vi "MecaKinematics_SetInverseKinematics.vi"(8 "RearRight":T2 {"Y" format="%14.3f"; "X" format="%14.3f"}, 9 "RearLeft":T2 {"Y" format="%14.3f"; "X" format="%14.3f"}, 10 "FrontRight":T2 {"Y" format="%14.3f"; "X" format="%14.3f"}, 11 "FrontLeft":T2 {"Y" format="%14.3f"; "X" format="%14.3f"}) -> (3 "InverseKinematics":T1)   [LabVIEW 2019, in "Trajectory_Library.lvlib"]
doc: "Construct inverse kinematics matrix from wheel locations.\n\nParameters:\n - FrontLeft - The location of the front-left wheel relative to the physical center of the robot.\n - FrontRight - The location of the front-right wheel relative to the physical center of the robot.\n - RearLeft - The location of the rear-left wheel relative to the physical center of the robot.\n - RearRight - The location of the rear-right wheel relative to the physical center of the robot.\n\nReturns:\n - InverseKinematics - Return matix"
uses:
  Trajectory_Library.lvlib
  TRANSLATION2D.ctl
  <vilib>/Analysis/Matrix/Datatypes/RealMatrix.ctl
  MatrixHelper_CoerceSize.vi
  <vilib>/Analysis/Matrix/NI_Matrix.lvlib
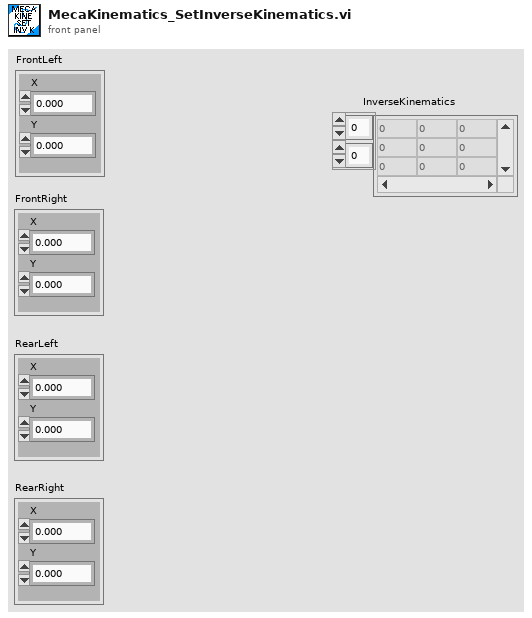
[diagram p1: front panel]
types:
  T1 = typedef "NI_Matrix.lvlib/RealMatrix.ctl" = dbl[][]
  T2 = typedef "Trajectory_Library.lvlib/TRANSLATION2D.ctl" = cluster{"X":dbl, "Y":dbl}
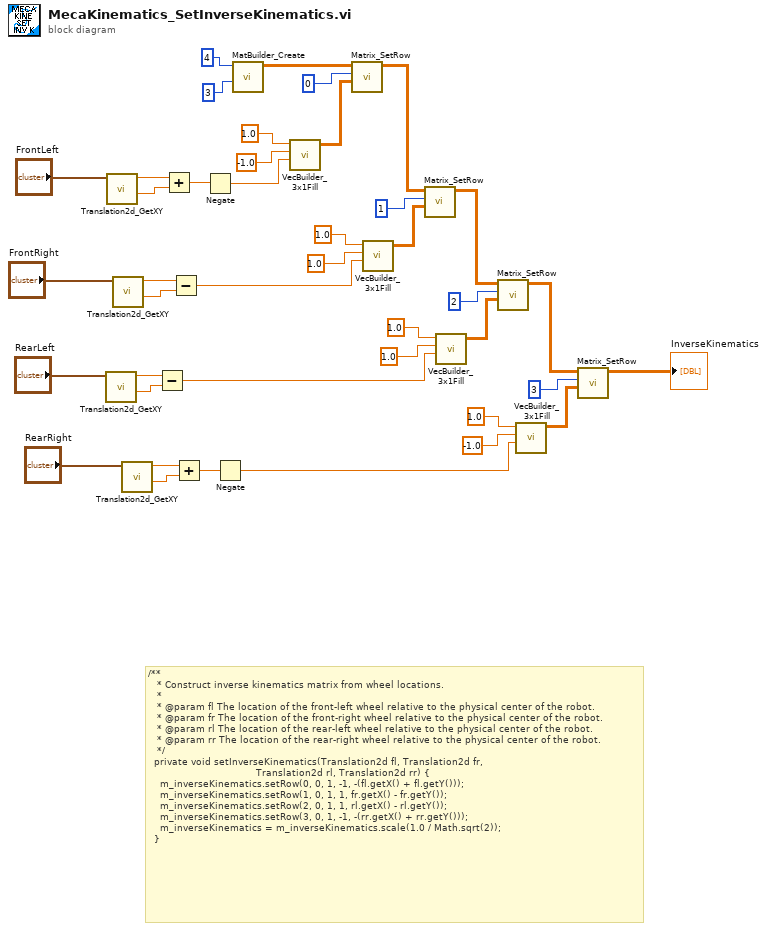
[diagram p0: block diagram]
diagram:
  # "/**\n   * Construct inverse kinematics matrix from wheel locations.\n   *\n   * @param fl The location of the front-left wheel relative to the physical center of the robot.\n   * @param fr The location of the front-right wheel relative to the physical center of the robot.\n   * @param rl The location of the rear-left wheel relative to the physical center of the robot.\n   * @param rr The location of the rear-right wheel relative to the physical center of the robot.\n   */\n  private void setInverseKinematics(Translation2d fl, Translation2d fr,\n                                    Translation2d rl, Translation2d rr) {\n    m_inverseKinematics.setRow(0, 0, 1, -1, -(fl.getX() + fl.getY()));\n    m_inverseKinematics.setRow(1, 0, 1, 1, fr.getX() - fr.getY());\n    m_inverseKinematics.setRow(2, 0, 1, 1, rl.getX() - rl.getY());\n    m_inverseKinematics.setRow(3, 0, 1, -1, -(rr.getX() + rr.getY()));\n    m_inverseKinematics = m_inverseKinematics.scale(1.0 / Math.sqrt(2));\n  }"
  n1 = call "Translation2d_GetXY.vi"("In Translation"="RearLeft") -> ("Y"=w4:dbl, "X"=w5:dbl)  [unwired: 9 in]
  n2 = call "Translation2d_GetXY.vi"("In Translation"="FrontLeft") -> ("Y"=w8:dbl, "X"=w9:dbl)  [unwired: 9 in]
  n3 = call "Translation2d_GetXY.vi"("In Translation"="FrontRight") -> ("Y"=w6:dbl, "X"=w7:dbl)  [unwired: 9 in]
  n4 = call "Translation2d_GetXY.vi"("In Translation"="RearRight") -> ("Y"=w2:dbl, "X"=w3:dbl)  [unwired: 9 in]
  n5 = Subtract(x=w5, y=w4) -> (x-y=w19:dbl)
  n6 = Add(x=w9, y=w8) -> (x+y=w41:dbl)
  n7 = Subtract(x=w7, y=w6) -> (x-y=w21:dbl)
  n8 = Add(x=w3, y=w2) -> (x+y=w40:dbl)
  n9 = Negate(x=w41) -> (-x=w36:dbl)
  n10 = Negate(x=w40) -> (-x=w14:dbl)
  n11 = call "MatBuilder_Create.vi"("Columns"=3, "Rows"=4) -> ("output matrix"=w16:T1)  [unwired: 9 in]
  n12 = call "VecBuilder_3x1Fill.vi"("R2"=w36, "R1"=-1.0, "R0"=1.0) -> ("output matrix"=w35:T1)  [unwired: 8 in]
  n13 = call "Matrix_SetRow.vi"("Fill Row Vector"=w35, "Row"=0, "input matrix"=w16) -> ("output matrix"=w22:T1)  [unwired: 7 in, 1 out]
  n14 = call "VecBuilder_3x1Fill.vi"("R2"=w21, "R1"=1.0, "R0"=1.0) -> ("output matrix"=w31:T1)  [unwired: 8 in]
  n15 = call "Matrix_SetRow.vi"("Fill Row Vector"=w31, "Row"=1, "input matrix"=w22) -> ("output matrix"=w20:T1)  [unwired: 7 in, 1 out]
  n16 = call "VecBuilder_3x1Fill.vi"("R2"=w19, "R1"=1.0, "R0"=1.0) -> ("output matrix"=w27:T1)  [unwired: 8 in]
  n17 = call "Matrix_SetRow.vi"("Fill Row Vector"=w27, "Row"=2, "input matrix"=w20) -> ("output matrix"=w15:T1)  [unwired: 7 in, 1 out]
  n18 = call "VecBuilder_3x1Fill.vi"("R2"=w14, "R1"=-1.0, "R0"=1.0) -> ("output matrix"=w23:T1)  [unwired: 8 in]
  n19 = call "Matrix_SetRow.vi"("Fill Row Vector"=w23, "Row"=3, "input matrix"=w15) -> ("output matrix"=→"InverseKinematics":T1)  [unwired: 7 in, 1 out]
